vi "STAV Programs read_write.vi"() -> ()   [LabVIEW 2021]
uses:
  Czytaj RS/Biblioteki/Statyw/Application.ctl
  Czytaj RS/Biblioteki/Statyw/STAV CommandList.ctl
  Czytaj RS/Biblioteki/Statyw/STAV lib.lvlib
panel:
  out "String":string
  in  "stop":bool
  in  "Tab Control":enum32{"Konfig", "Page 2", "Help", "Debug"}(tab)
  in  "STAV com port":refnum<visa-resource-name>="COM4"
  in  "Refresh":bool
  in  "Set Active":bool
  in  "Dane":i32(listbox)
  in  "Pobierz":bool
  in  "NO":u8=1 min=1 max=50 step=1
  in  "Application":T1
  in  "Run app":bool
  in  "Stop app":bool
  in  "Reset app":bool
  in  "check active":bool
  out "Profile":string
  out "Steps":i32
  out "Step":string
  # "Units: Metric, Imperial"
  # "Direction: Up, Down"
  # "Mode: Cycles, Time"
  # "Stop Condition:\nDuration, Distance, Position, F greater, F smaller, Break, Keep F"
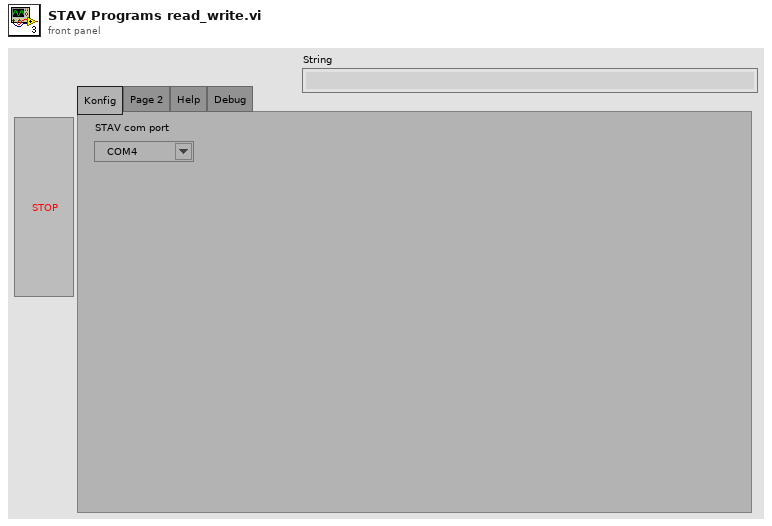
[diagram p1: front panel]
types:
  T1 = typedef "STAV lib.lvlib/Application.ctl" = enum16{"Peak", "Cycle", "Step", "Advanced"}
  T2 = enum8{"Enabled", "Disabled", "Disabled and Grayed Out"}
  T3 = typedef "STAV lib.lvlib/STAV CommandList.ctl" = enum16{"StartSending (0)", "StopSending(0)", "FindHomePos(0)", "SetSendingConfig(2)", "GetSendingConfig(0)", "SetPosition(2)", "SetSpeed(2)", "GetSpeed(0)", "GetPosition(0)", "GetForce(0)", "GetPeak(0)", "GetPeakDistance(0)", "GetTravelDistance(0)", "ResetTravelDistance(0)", "GetCycleNo(0)", "GetStepNo(0)", "GetDuration(0)", "GetProfilePosition(0)", "GetHoldTime(0)", "Stop(0)", "StartAndSend(0)", "Start(0)", "Reset(0)", "GetActiveProfile(0)", "SetActiveProfile(2)", "GetProfileCnt(1)", "GetMaxStepCnt(1)", "GetStepCnt(2)", "GetProfileIndex(2)", "SetProfile(3)", "SetStep(3+params)", "GetProfile(2)", "GetStep(3)", "SetProfile(2+params)", ""}
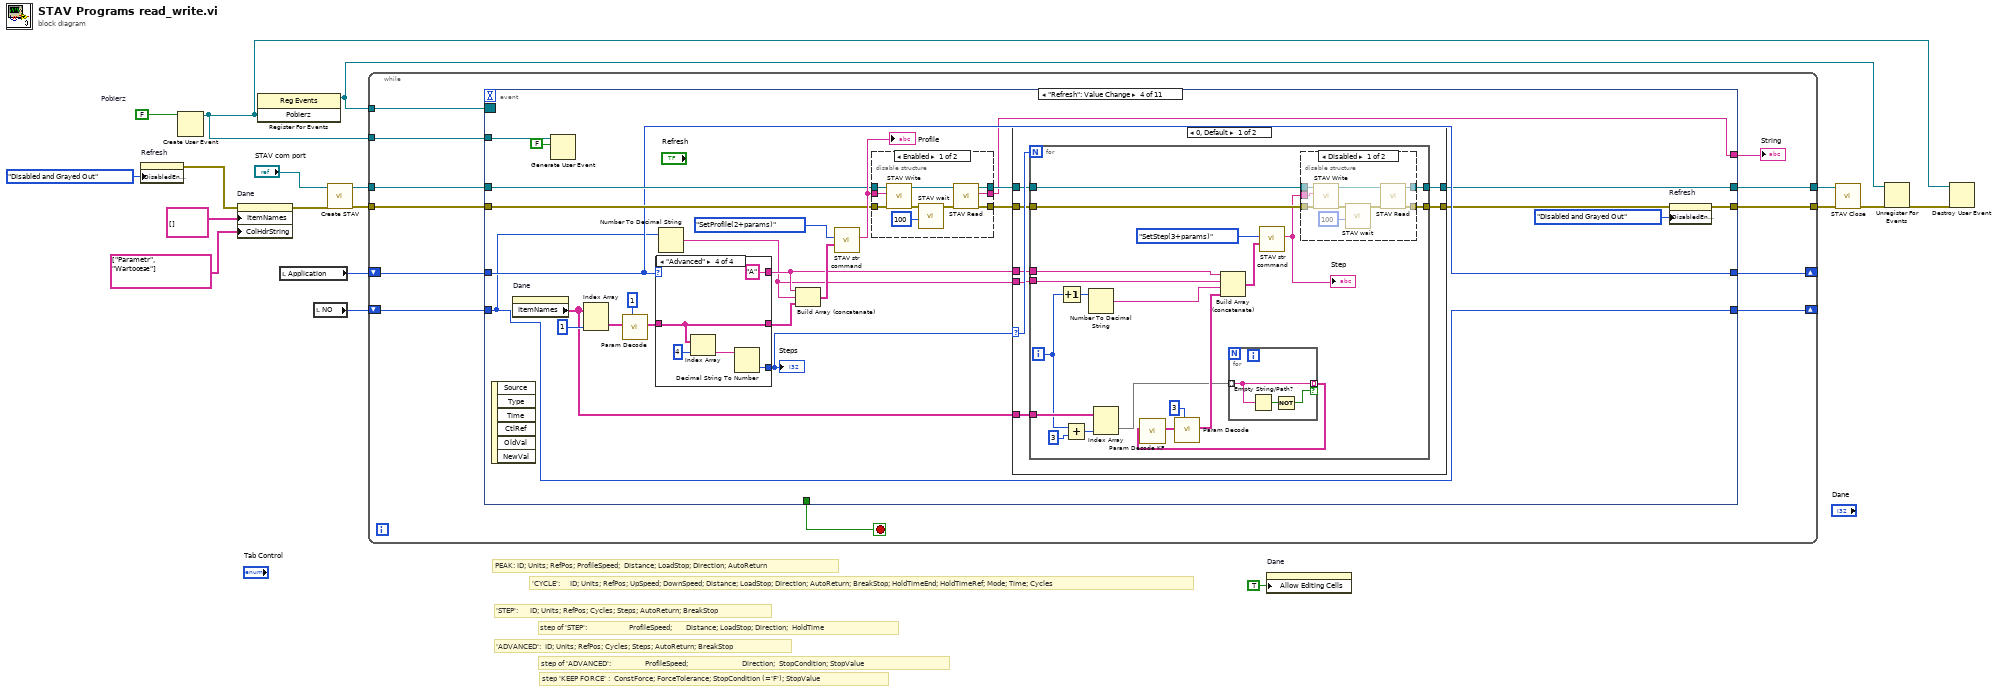
[diagram p0: block diagram]
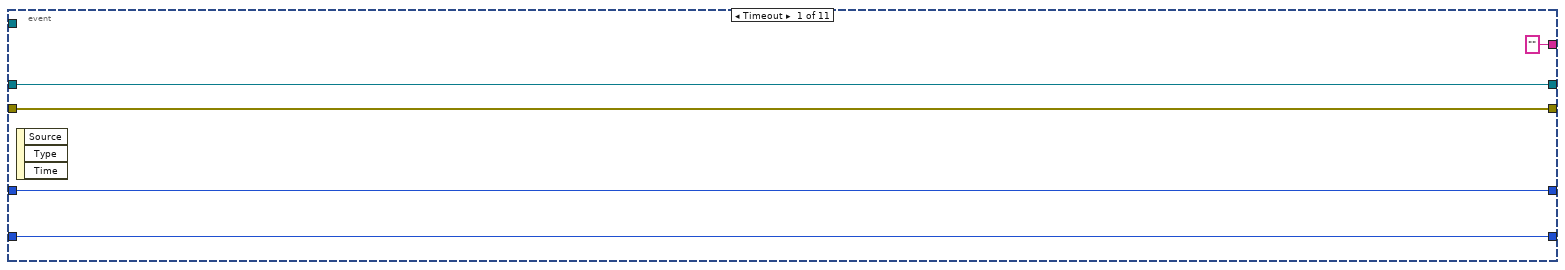
[diagram p2: hidden frame]
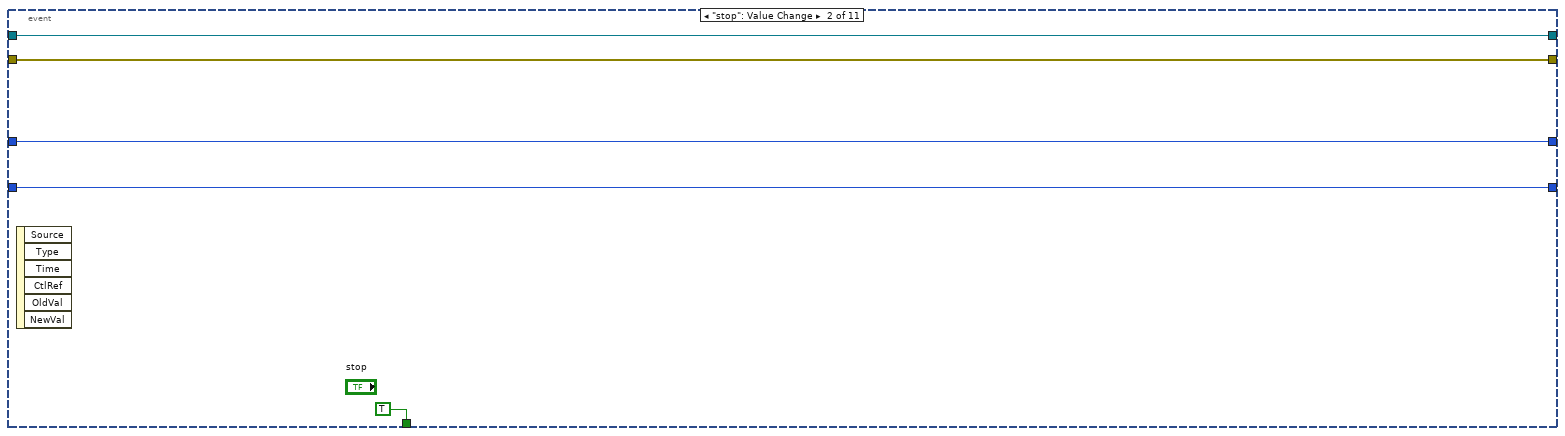
[diagram p3: hidden frame]
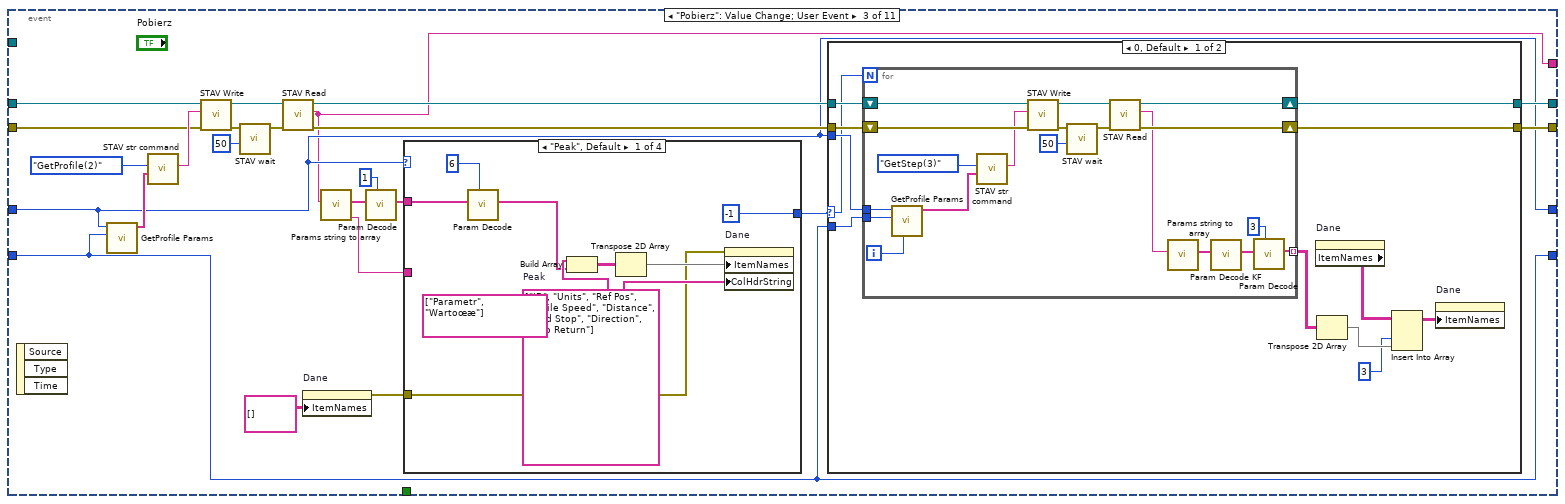
[diagram p4: hidden frame]
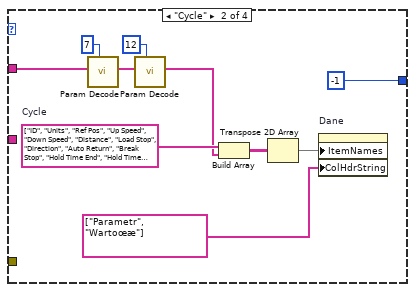
[diagram p6: hidden frame]
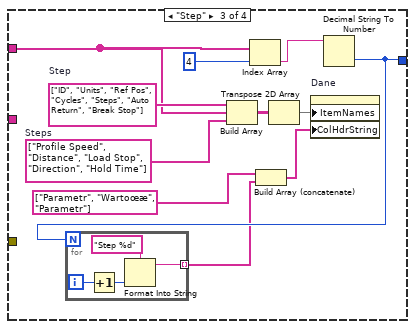
[diagram p7: hidden frame]
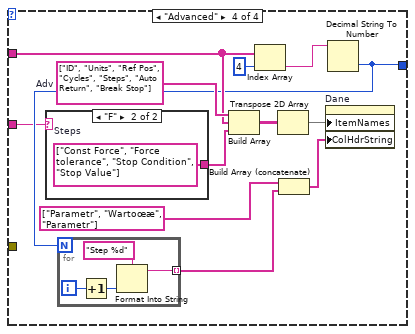
[diagram p8: hidden frame]
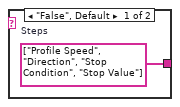
[diagram p9: hidden frame]
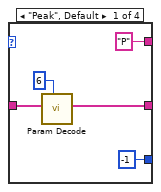
[diagram p13: hidden frame]
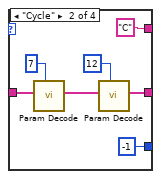
[diagram p14: hidden frame]
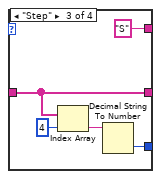
[diagram p15: hidden frame]
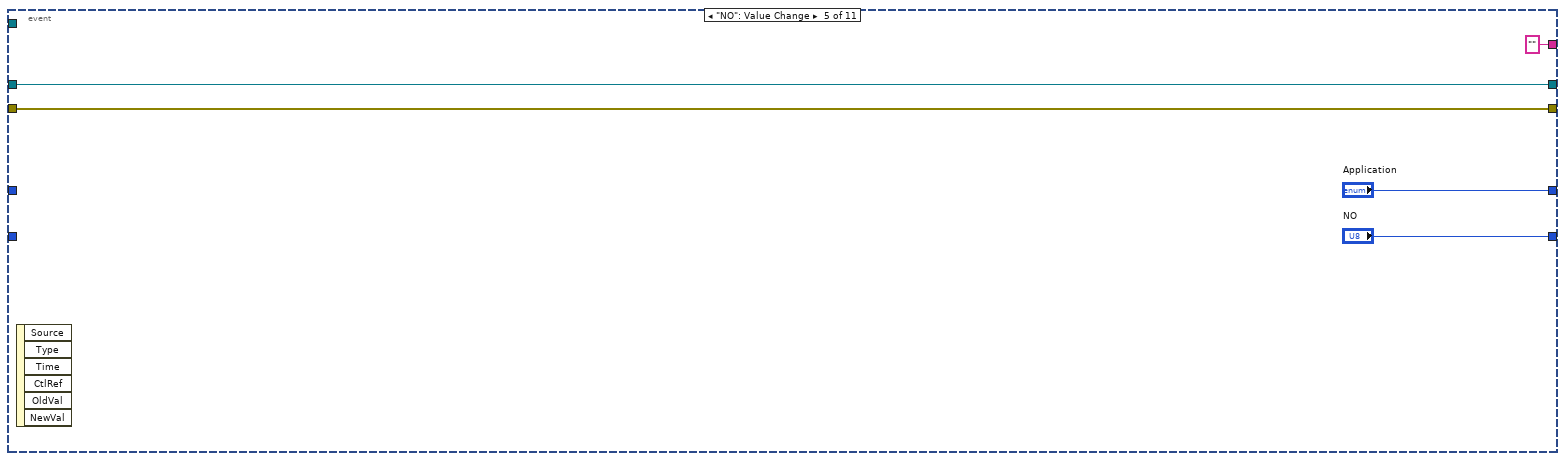
[diagram p16: hidden frame]
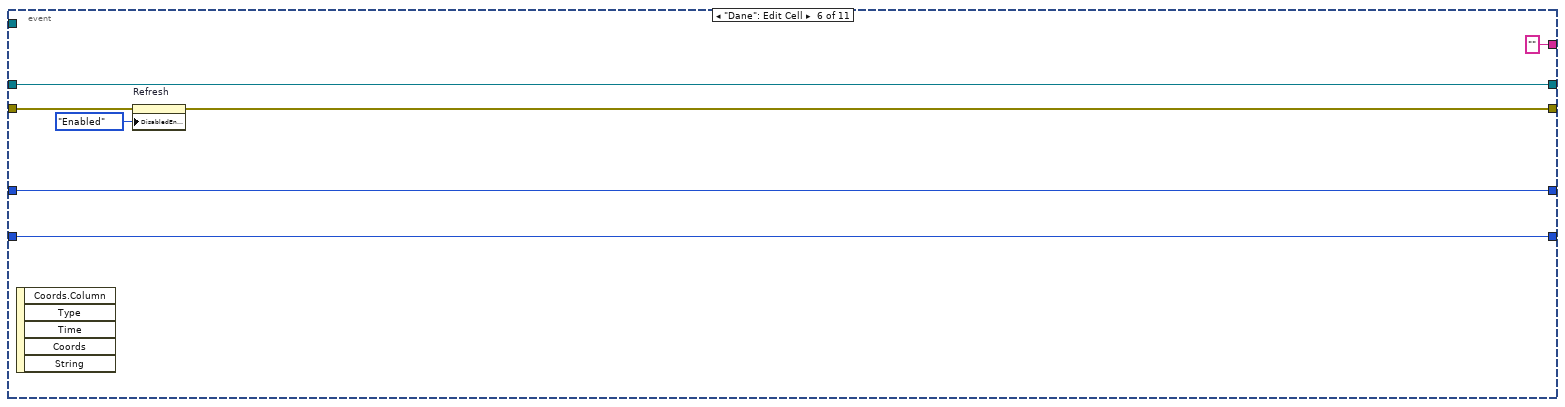
[diagram p17: hidden frame]
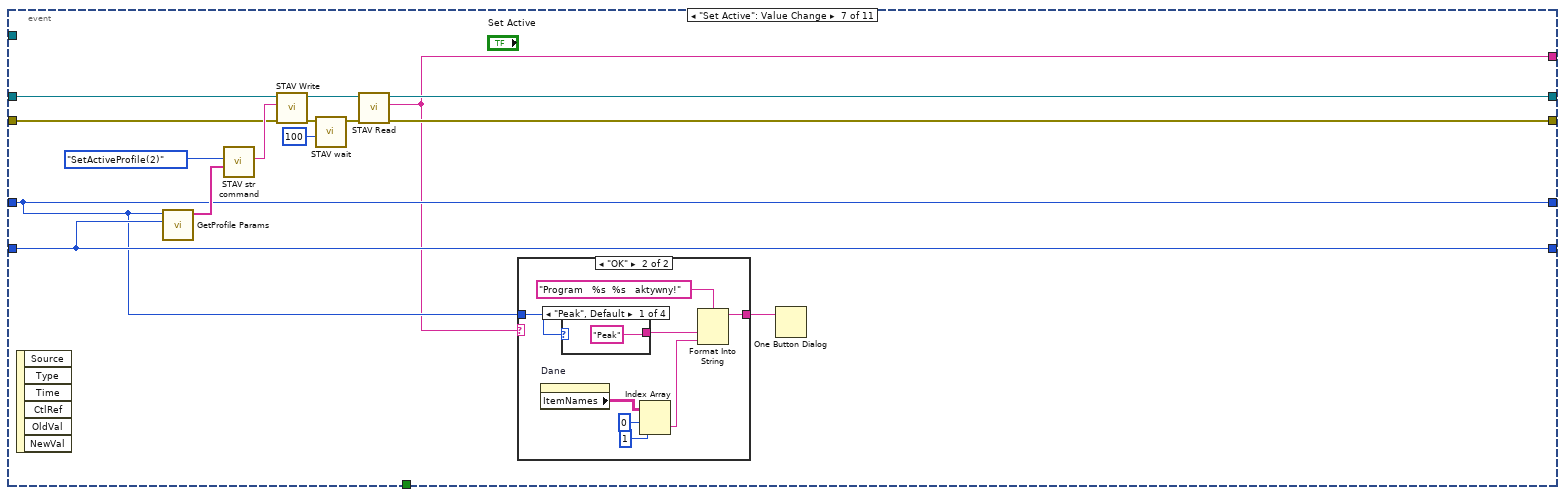
[diagram p18: hidden frame]
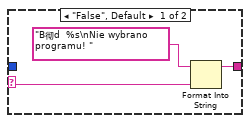
[diagram p19: hidden frame]
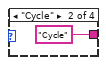
[diagram p20: hidden frame]
diagram:
  w5 = FALSE  # Pobierz
  # "step 'KEEP FORCE' :  ConstForce; ForceTolerance; StopCondition (='F'); StopValue"
  # "step of 'ADVANCED':                 ProfileSpeed;                           Direction;  StopCondition; StopValue"
  # "'ADVANCED':  ID; Units; RefPos; Cycles; Steps; AutoReturn; BreakStop"
  # "step of 'STEP':                     ProfileSpeed;       Distance; LoadStop; Direction;  HoldTime"
  # "'STEP':      ID; Units; RefPos; Cycles; Steps; AutoReturn; BreakStop"
  # "'CYCLE':     ID; Units; RefPos; UpSpeed; DownSpeed; Distance; LoadStop; Direction; AutoReturn; BreakStop; HoldTimeEnd; HoldTimeRef; Mode; Time; Cycles"
  # "PEAK: ID; Units; RefPos; ProfileSpeed;  Distance; LoadStop; Direction; AutoReturn"
  n1 = property on="Refresh" class="Bool"("DisabledEnum"=T2."Disabled and Grayed Out" ("Disabled")) -> (error out=w9:errorcluster)  [unwired: 2 in, 1 out]
  n2 = Create User Event(user event datatype=w5) -> (user event=w3:refnum<user-event>)  [unwired: 1 in, 1 out]
  n3 = property on="Dane" class="MCListbox (strict)"(error in=w9, "ItemNames"=string[][] [] ("Item Names"), "ColHdrString"=string[] ["Parametr", "Wartoœæ"] ("Column Header Strings[]")) -> (error out=w12:errorcluster)  [unwired: 1 in, 1 out]
  n4 = register-events(w3) -> (reference out=w4:refnum<event-registration>)  [unwired: 2 in, 1 out]
  n5 = local read "Application"() -> (w7:T1)
  n6 = local read "NO"() -> (w6:u8)
  n7 = call "Create STAV.vi"("error in (no error)"=w12, "STAV com port"="STAV com port") -> ("error out"=w16:errorcluster, "STAV ref out"=w17:refnum<visa-resource-name>)  [unwired: 8 in]
  n8 = while {
    tunnel: w17 -> [w29]
    tunnel: w16 -> [w28]
    tunnel: [w27] -> w15
    tunnel: [w26] -> w14
    shift-right: [w25] -> _
    shift-left: w7 -> [w23]
    shift-right: [w24] -> _
    shift-left: w6 -> [w22]
    tunnel: w4 -> [w21]
    tunnel: w3 -> [w20]
    stop <- w30 stop-if-true
    n9 = event shown="[3] \"Refresh\": Value Change" {
      selector: w21 -> [_ _ _ _ _ _ _ _ _ _ _]
      dyn-events: _ -> [_ _ _ _ _ _ _ _ _ _ _]
      timeout: _ -> [_ _ _ _ _ _ _ _ _ _ _]
      tunnel: [_ TRUE ("stop") _ _ _ _ _ _ _ _ _] -> w30
      tunnel: w29 -> [w35 w39 w61 w170 w252 w260 w270 w307 w330 w343 w356]
      tunnel: w28 -> [w34 w38 w60 w171 w253 w262 w271 w308 w329 w342 w355]
      tunnel: [w35 w39 w52 w155 w252 w260 w267 w304 w326 w339 w352] -> w27
      tunnel: [w34 w38 w50 w160 w253 w261 w268 w305 w327 w340 w353] -> w26
      tunnel: w22 -> [w32 w36 w45 w167 _ w258 w269 w306 w331 w344 w357]
      tunnel: w23 -> [w33 w37 w44 w168 _ w259 w265 w303 w332 w345 w358]
      tunnel: [w33 w37 w44 w168 "Application" w259 w265 w303 w332 w345 w358] -> w25
      tunnel: [w32 w36 w45 w167 "NO" w258 w269 w306 w331 w344 w357] -> w24
      tunnel: w20 -> [_ _ _ w151 _ _ _ _ _ _ _]
      tunnel: ["" ("String") _ w41 w149 "" ("String") "" ("String") w264 w294 w320 w333 w346] -> w19
      event Timeout {
        n10 = event-data() -> ()  [unwired: 1 in, 3 out]
      }
      event "stop": Value Change {
        n11 = event-data() -> ()  [unwired: 1 in, 6 out]
      }
      event "Pobierz": Value Change; User Event {
        n12 = event-data() -> ()  [unwired: 1 in, 3 out]
        n13 = call "GetProfile Params.vi"("NO"=w45, "Application"=w44) -> ("params array out"=w57:string[])  [unwired: 7 in, 2 out]
        n14 = call "STAV str command.vi"("Params"=w57, "Command"=STAV_CommandList."GetProfile(2)") -> ("str command"=w63:string)  [unwired: 8 in, 1 out]
        n15 = call "STAV Write.vi"("error in (no error)"=w60, "Command"=w63, "STAV ref in"=w61) -> ("error out"=w58:errorcluster, "STAV ref out"=w59:refnum<visa-resource-name>)  [unwired: 7 in]
        n16 = call "STAV wait.vi"("delay (20)"=u32 50, "error in (no error)"=w58) -> ("error out"=w56:errorcluster)  [unwired: 9 in]
        n17 = call "STAV Read.vi"("error in (no error)"=w56, "STAV ref in"=w59) -> ("error out"=w51:errorcluster, "String"=w41:string, "STAV ref out"=w53:refnum<visa-resource-name>)  [unwired: 6 in, 1 out]
        n18 = property on="Dane" class="MCListbox (strict)"("ItemNames"=string[][] [] ("Item Names")) -> (error out=w42:errorcluster)  [unwired: 2 in, 1 out]
        n19 = call "Params string to array.vi"("String params"=w41) -> ("Last"=w49:string, "Array of params"=w47:string[])  [unwired: 9 in]
        n20 = call "Param Decode.vi"("index"=1, "Array - letter"=w47) -> ("Array -parameter"=w46:string[])  [unwired: 8 in, 1 out]
        n21 = case shown="\"Peak\", Default" w44 {
          tunnel: w46 -> [w100 w110 w116 w138]
          tunnel: [-1 -1 w119 w135] -> w54
          tunnel: w49 -> [_ _ _ w131]
          tunnel: w42 -> [w97 _ _ _]
          frame "Peak", Default {
            w105 = string[] ["ID", "Units", "Ref Pos", "Profile Speed", "Distance", "Load Stop", "Direction", "Auto Return"]  # Peak
            n22 = call "Param Decode.vi"("index"=6, "Array - letter"=w100) -> ("Array -parameter"=w99:string[])  [unwired: 8 in, 1 out]
            n23 = Build Array(w105, w99) -> (w104:string[][])
            n24 = Transpose 2D Array(2D array=w104) -> (transposed array=w103:string[][])
            n25 = property on="Dane" class="MCListbox (strict)"(error in=w97, "ItemNames"=w103, "ColHdrString"=string[] ["Parametr", "Wartoœæ"] ("Column Header Strings[]")) -> ()  [unwired: 1 in, 2 out]
          }
          frame "Cycle" {
            w114 = string[] ["ID", "Units", "Ref Pos", "Up Speed", "Down Speed", "Distance", "Load Stop", "Direction", "Auto Return", "Break Stop", "Hold Time End", "Hold Time Ref", "Mode", "Time", "Cycles"]  # Cycle
            n26 = call "Param Decode.vi"("index"=7, "Array - letter"=w110) -> ("Array -parameter"=w107:string[])  [unwired: 8 in, 1 out]
            n27 = call "Param Decode.vi"("index"=12, "Array - letter"=w107) -> ("Array -parameter"=w106:string[])  [unwired: 8 in, 1 out]
            n28 = Build Array(w114, w106) -> (w115:string[][])
            n29 = Transpose 2D Array(2D array=w115) -> (transposed array=w113:string[][])
            n30 = property on="Dane" class="MCListbox (strict)"("ItemNames"=w113, "ColHdrString"=string[] ["Parametr", "Wartoœæ"] ("Column Header Strings[]")) -> ()  [unwired: 2 in, 2 out]
          }
          frame "Step" {
            w117 = string[] ["Profile Speed", "Distance", "Load Stop", "Direction", "Hold Time"]  # Steps
            w124 = string[] ["ID", "Units", "Ref Pos", "Cycles", "Steps", "Auto Return", "Break Stop"]  # Step
            n31 = Build Array(w124, w116, w117) -> (w126:string[][])
            n32 = Index Array(array=w116, index=4) -> (element=w122:string)
            n33 = Transpose 2D Array(2D array=w126) -> (transposed array=w125:string[][])
            n34 = Decimal String To Number(string=w122) -> (number=w119:i32)  [unwired: 2 in, 1 out]
            n35 = for {
              N: w119 -> [_]
              tunnel: [w128] -> w118 mode=indexing
              i -> [w130]
              n36 = Increment(x=w130) -> (x+1=w127:i32)
              n37 = Format Into String(format string="Step %d", w127) -> (resulting string=w128:string)  [unwired: 2 in, 1 out]
            }
            n38 = Build Array (concatenate)(string[] ["Parametr", "Wartoœæ", "Parametr"] ("Column Header Strings[]"), w118) -> (w120:string[])
            n39 = property on="Dane" class="MCListbox (strict)"("ItemNames"=w125, "ColHdrString"=w120) -> ()  [unwired: 2 in, 2 out]
          }
          frame "Advanced" {
            w139 = string[] ["ID", "Units", "Ref Pos", "Cycles", "Steps", "Auto Return", "Break Stop"]  # Adv
            n40 = case shown="\"F\"" w131 {
              tunnel: [w143 w144] -> w132
              frame "False", Default {
                w143 = string[] ["Profile Speed", "Direction", "Stop Condition", "Stop Value"]  # Steps
              }
              frame "F" {
                w144 = string[] ["Const Force", "Force tolerance", "Stop Condition", "Stop Value"]  # Steps
              }
            }
            n41 = Build Array(w139, w138, w132) -> (w142:string[][])
            n42 = Index Array(array=w138, index=4) -> (element=w136:string)
            n43 = Transpose 2D Array(2D array=w142) -> (transposed array=w141:string[][])
            n44 = Decimal String To Number(string=w136) -> (number=w135:i32)  [unwired: 2 in, 1 out]
            n45 = for {
              N: w135 -> [_]
              tunnel: [w146] -> w133 mode=indexing
              i -> [w148]
              n46 = Increment(x=w148) -> (x+1=w145:i32)
              n47 = Format Into String(format string="Step %d", w145) -> (resulting string=w146:string)  [unwired: 2 in, 1 out]
            }
            n48 = Build Array (concatenate)(string[] ["Parametr", "Wartoœæ", "Parametr"] ("Column Header Strings[]"), w133) -> (w134:string[])
            n49 = property on="Dane" class="MCListbox (strict)"("ItemNames"=w141, "ColHdrString"=w134) -> ()  [unwired: 2 in, 2 out]
          }
        }
        n50 = case shown="0, Default" w54 {
          selector: w54 -> [w69 _]
          tunnel: w53 -> [w74 w96]
          tunnel: [w72 w96] -> w52
          tunnel: w51 -> [w75 w95]
          tunnel: [w73 w95] -> w50
          tunnel: w44 -> [w71 _]
          tunnel: w45 -> [w70 _]
          frame 0, Default {
            n51 = for {
              N: w69 -> [_]
              shift-right: [w87] -> w73
              shift-left: w75 -> [w89]
              shift-right: [w86] -> w72
              shift-left: w74 -> [w88]
              tunnel: w71 -> [w84]
              tunnel: w70 -> [w83]
              tunnel: [w78] -> w68 mode=indexing
              i -> [w80]
              n52 = call "GetProfile Params.vi"("Step (-1)"=w80, "NO"=w83, "Application"=w84) -> ("params array out"=w82:string[])  [unwired: 6 in, 2 out]
              n53 = call "STAV str command.vi"("Params"=w82, "Command"=STAV_CommandList."GetStep(3)") -> ("str command"=w85:string)  [unwired: 8 in, 1 out]
              n54 = call "STAV Write.vi"("error in (no error)"=w89, "Command"=w85, "STAV ref in"=w88) -> ("error out"=w91:errorcluster, "STAV ref out"=w90:refnum<visa-resource-name>)  [unwired: 7 in]
              n55 = call "STAV wait.vi"("delay (20)"=u32 50, "error in (no error)"=w91) -> ("error out"=w92:errorcluster)  [unwired: 9 in]
              n56 = call "STAV Read.vi"("error in (no error)"=w92, "STAV ref in"=w90) -> ("error out"=w87:errorcluster, "String"=w81:string, "STAV ref out"=w86:refnum<visa-resource-name>)  [unwired: 6 in, 1 out]
              n57 = call "Params string to array.vi"("String params"=w81) -> ("Array of params"=w77:string[])  [unwired: 9 in, 1 out]
              n58 = call "Param Decode KF.vi"("Array - letter"=w77) -> ("Array -parameter"=w76:string[])  [unwired: 9 in, 1 out]
              n59 = call "Param Decode.vi"("index"=3, "Array - letter"=w76) -> ("Array -parameter"=w78:string[])  [unwired: 8 in, 1 out]
            }
            n60 = property on="Dane" class="MCListbox (strict)"() -> ("ItemNames"=w67:string[][])  [unwired: 2 in, 2 out]
            n61 = Transpose 2D Array(2D array=w68) -> (transposed array=w65:string[][])
            n62 = Insert Into Array(array=w67, index (col)=3 ("disabled index (col)"), new element=w65) -> (w66:string[][])  [unwired: 1 in]
            n63 = property on="Dane" class="MCListbox (strict)"("ItemNames"=w66) -> ()  [unwired: 2 in, 2 out]
          }
          frame -1 {
          }
        }
      }
      event "Refresh": Value Change {
        n64 = event-data() -> ()  [unwired: 1 in, 6 out]
        n65 = property on="Dane" class="MCListbox (strict)"() -> ("ItemNames"=w154:string[][])  [unwired: 2 in, 2 out]
        n66 = Generate User Event(user event=w151, event data cluster=FALSE ("event data")) -> ()  [unwired: 2 in, 2 out]
        n67 = Index Array(array=w154, index (col)=1 ("disabled index (col)")) -> (element=w164:string[])  [unwired: 1 in]
        n68 = call "Param Decode.vi"("index"=1, "Array - letter"=w164) -> ("Array -parameter"=w163:string[])  [unwired: 8 in, 1 out]
        n69 = case shown="\"Advanced\"" w168 {
          tunnel: ["P" "C" "S" "A"] -> w153
          tunnel: w163 -> [w233 w240 w245 w249]
          tunnel: [w232 w237 w245 w249] -> w165
          tunnel: [-1 -1 w242 w247] -> w159
          frame "Peak", Default {
            n70 = call "Param Decode.vi"("index"=6, "Array - letter"=w233) -> ("Array -parameter"=w232:string[])  [unwired: 8 in, 1 out]
          }
          frame "Cycle" {
            n71 = call "Param Decode.vi"("index"=7, "Array - letter"=w240) -> ("Array -parameter"=w238:string[])  [unwired: 8 in, 1 out]
            n72 = call "Param Decode.vi"("index"=12, "Array - letter"=w238) -> ("Array -parameter"=w237:string[])  [unwired: 8 in, 1 out]
          }
          frame "Step" {
            n73 = Index Array(array=w245, index=4) -> (element=w243:string)
            n74 = Decimal String To Number(string=w243) -> (number=w242:i32)  [unwired: 2 in, 1 out]
          }
          frame "Advanced" {
            n75 = Index Array(array=w249, index=4) -> (element=w248:string)
            n76 = Decimal String To Number(string=w248) -> (number=w247:i32)  [unwired: 2 in, 1 out]
          }
        }
        "Steps" <- w159
        n77 = Number To Decimal String(number=w167) -> (decimal integer string=w152:string)  [unwired: 1 in]
        n78 = Build Array (concatenate)(w153, w152, w165) -> (w166:string[])
        n79 = call "STAV str command.vi"("Params"=w166, "Command"=STAV_CommandList."SetProfile(2+params)") -> ("str command"=w173:string)  [unwired: 8 in, 1 out]
        "Profile" <- w173
        n80 = disable-structure shown="Enabled" {
          disable-tunnel: w173 -> [w227 _]
          disable-tunnel: w171 -> [w222 w228]
          disable-tunnel: w170 -> [w221 w229]
          disable-tunnel: [w220 w228] -> w157
          disable-tunnel: [w219 w229] -> w158
          disable-tunnel: [w218 _] -> w149
          frame Enabled {
            n81 = call "STAV Write.vi"("error in (no error)"=w222, "Command"=w227, "STAV ref in"=w221) -> ("error out"=w225:errorcluster, "STAV ref out"=w226:refnum<visa-resource-name>)  [unwired: 7 in]
            n82 = call "STAV wait.vi"("delay (20)"=u32 100, "error in (no error)"=w225) -> ("error out"=w224:errorcluster)  [unwired: 9 in]
            n83 = call "STAV Read.vi"("error in (no error)"=w224, "STAV ref in"=w226) -> ("error out"=w220:errorcluster, "String"=w218:string, "STAV ref out"=w219:refnum<visa-resource-name>)  [unwired: 6 in, 1 out]
          }
          frame Disabled {
          }
        }
        n84 = case shown="0, Default" w159 {
          selector: w159 -> [w181 _]
          tunnel: w158 -> [w180 w216]
          tunnel: w157 -> [w179 w217]
          tunnel: [w178 w217] -> w156
          tunnel: [w177 w216] -> w155
          tunnel: w154 -> [w176 _]
          tunnel: w153 -> [w175 _]
          tunnel: w152 -> [w174 _]
          frame 0, Default {
            n85 = for {
              N: w181 -> [_]
              tunnel: w180 -> [w200]
              tunnel: w179 -> [w199]
              tunnel: [w198] -> w178
              tunnel: [w197] -> w177
              tunnel: w176 -> [w196]
              tunnel: w175 -> [w195]
              tunnel: w174 -> [w194]
              i -> [w191]
              n86 = Increment(x=w191) -> (x+1=w193:i32)
              n87 = Add(x=w191, y=3) -> (x+y=w184:i32)
              n88 = Number To Decimal String(number=w193) -> (decimal integer string=w192:string)  [unwired: 1 in]
              n89 = Index Array(array=w196, index (col)=w184) -> (element=w183:string[])  [unwired: 1 in]
              n90 = for {
                tunnel: w183 -> [w204] mode=indexing
                tunnel: [w204] -> w182 mode=indexing if=w202
                n91 = Empty String/Path?(string/path=w204) -> (empty?=w203:bool)
                n92 = Not(x=w203) -> (.not. x?=w202:bool)
              }
              n93 = call "Param Decode KF.vi"("Array - letter"=w182) -> ("Array -parameter"=w186:string[])  [unwired: 9 in, 1 out]
              n94 = call "Param Decode.vi"("index"=3, "Array - letter"=w186) -> ("Array -parameter"=w185:string[])  [unwired: 8 in, 1 out]
              n95 = Build Array (concatenate)(w195, w194, w192, w185) -> (w189:string[])
              n96 = call "STAV str command.vi"("Params"=w189, "Command"=STAV_CommandList."SetStep(3+params)") -> ("str command"=w188:string)  [unwired: 8 in, 1 out]
              "Step" <- w188
              n97 = disable-structure shown="Disabled" {
                disable-tunnel: w200 -> [w209 w215]
                disable-tunnel: w199 -> [w208 w214]
                disable-tunnel: [w207 w214] -> w198
                disable-tunnel: [w206 w215] -> w197
                disable-tunnel: w188 -> [w205 _]
                frame Disabled {
                  n98 = call "STAV Write.vi"("error in (no error)"=w208, "Command"=w205, "STAV ref in"=w209) -> ("error out"=w211:errorcluster, "STAV ref out"=w210:refnum<visa-resource-name>)  [unwired: 7 in]
                  n99 = call "STAV wait.vi"("delay (20)"=u32 100, "error in (no error)"=w211) -> ("error out"=w212:errorcluster)  [unwired: 9 in]
                  n100 = call "STAV Read.vi"("error in (no error)"=w212, "STAV ref in"=w210) -> ("error out"=w207:errorcluster, "STAV ref out"=w206:refnum<visa-resource-name>)  [unwired: 6 in, 2 out]
                }
                frame Enabled {
                }
              }
            }
          }
          frame -1 {
          }
        }
        n101 = property on="Refresh" class="Bool"(error in=w156, "DisabledEnum"=T2."Disabled and Grayed Out" ("Disabled")) -> (error out=w160:errorcluster)  [unwired: 1 in, 1 out]
      }
      event "NO": Value Change {
        n102 = event-data() -> ()  [unwired: 1 in, 6 out]
      }
      event "Dane": Edit Cell {
        n103 = event-data() -> ()  [unwired: 1 in, 5 out]
        n104 = property on="Refresh" class="Bool"(error in=w262, "DisabledEnum"=T2."Enabled" ("Disabled")) -> (error out=w261:errorcluster)  [unwired: 1 in, 1 out]
      }
      event "Set Active": Value Change {
        n105 = event-data() -> ()  [unwired: 1 in, 6 out]
        n106 = call "GetProfile Params.vi"("NO"=w269, "Application"=w265) -> ("params array out"=w274:string[])  [unwired: 7 in, 2 out]
        n107 = call "STAV str command.vi"("Params"=w274, "Command"=STAV_CommandList."SetActiveProfile(2)") -> ("str command"=w278:string)  [unwired: 8 in, 1 out]
        n108 = call "STAV Write.vi"("error in (no error)"=w271, "Command"=w278, "STAV ref in"=w270) -> ("error out"=w275:errorcluster, "STAV ref out"=w276:refnum<visa-resource-name>)  [unwired: 7 in]
        n109 = call "STAV wait.vi"("delay (20)"=u32 100, "error in (no error)"=w275) -> ("error out"=w273:errorcluster)  [unwired: 9 in]
        n110 = call "STAV Read.vi"("error in (no error)"=w273, "STAV ref in"=w276) -> ("error out"=w268:errorcluster, "String"=w264:string, "STAV ref out"=w267:refnum<visa-resource-name>)  [unwired: 6 in, 1 out]
        n111 = case shown="\"OK\"" w264 {
          selector: w264 -> [w280 _]
          tunnel: [w279 w285] -> w266
          tunnel: w265 -> [_ w284]
          frame "False", Default {
            n112 = Format Into String(initial string="B彻d  %s\nNie wybrano programu! ", w280) -> (resulting string=w279:string)  [unwired: 2 in, 1 out]
          }
          frame "OK" {
            n113 = property on="Dane" class="MCListbox (strict)"() -> ("ItemNames"=w289:string[][])  [unwired: 2 in, 2 out]
            n114 = case shown="\"Peak\", Default" w284 {
              tunnel: ["Peak" ("format string") "Cycle" ("format string") "Step" ("format string") "Advanced" ("format string")] -> w282
              frame "Peak", Default {
              }
              frame "Cycle" {
              }
              frame "Step" {
              }
              frame "Advanced" {
              }
            }
            n115 = Index Array(array=w289, index (row)=0, index (col)=1 ("disabled index (col)")) -> (element=w283:string)
            n116 = Format Into String(format string="Program   %s  %s   aktywny!", w282, w283) -> (resulting string=w285:string)  [unwired: 2 in, 1 out]
          }
        }
        n117 = One Button Dialog(message=w266) -> ()  [unwired: 1 in, 1 out]
      }
      event "check active": Value Change {
        n118 = event-data() -> ()  [unwired: 1 in, 6 out]
        n119 = call "STAV str command.vi"("Command"=STAV_CommandList."GetActiveProfile(0)") -> ("str command"=w314:string)  [unwired: 9 in, 1 out]
        n120 = call "STAV Write.vi"("error in (no error)"=w308, "Command"=w314, "STAV ref in"=w307) -> ("error out"=w311:errorcluster, "STAV ref out"=w312:refnum<visa-resource-name>)  [unwired: 7 in]
        n121 = call "STAV wait.vi"("delay (20)"=u32 100, "error in (no error)"=w311) -> ("error out"=w310:errorcluster)  [unwired: 9 in]
        n122 = call "STAV Read.vi"("error in (no error)"=w310, "STAV ref in"=w312) -> ("error out"=w305:errorcluster, "String"=w294:string, "STAV ref out"=w304:refnum<visa-resource-name>)  [unwired: 6 in, 1 out]
        n123 = String Subset(string=w294, offset (0)=0, length (rest)=1 ("length (rest)")) -> (substring=w299:string)
        n124 = String Subset(string=w294, offset (0)=2) -> (substring=w295:string)  [unwired: 1 in]
        n125 = case shown="\"False\", Default" w299 {
          tunnel: ["- brak -" ("substring") "Peak" ("substring") "Cycle" ("substring") "Step" ("substring") "Advanced" ("substring")] -> w296
          frame "False", Default {
          }
          frame "P" {
          }
          frame "C" {
          }
          frame "S" {
          }
          frame "A" {
          }
        }
        n126 = Format Into String(format string="Aktywny program \\n\n%s , numer %s", w296, w295) -> (resulting string=w297:string)  [unwired: 2 in, 1 out]
        n127 = One Button Dialog(message=w297) -> ()  [unwired: 1 in, 1 out]
      }
      event "Run app": Value Change {
        n128 = event-data() -> ()  [unwired: 1 in, 6 out]
        n129 = call "STAV str command.vi"("Command"=STAV_CommandList."Start(0)") -> ("str command"=w322:string)  [unwired: 9 in, 1 out]
        n130 = call "STAV Write.vi"("error in (no error)"=w329, "Command"=w322, "STAV ref in"=w330) -> ("error out"=w325:errorcluster, "STAV ref out"=w328:refnum<visa-resource-name>)  [unwired: 7 in]
        n131 = call "STAV wait.vi"("delay (20)"=u32 100, "error in (no error)"=w325) -> ("error out"=w324:errorcluster)  [unwired: 9 in]
        n132 = call "STAV Read.vi"("error in (no error)"=w324, "STAV ref in"=w328) -> ("error out"=w327:errorcluster, "String"=w320:string, "STAV ref out"=w326:refnum<visa-resource-name>)  [unwired: 6 in, 1 out]
      }
      event "Stop app": Value Change {
        n133 = event-data() -> ()  [unwired: 1 in, 6 out]
        n134 = call "STAV str command.vi"("Command"=STAV_CommandList."Stop(0)") -> ("str command"=w335:string)  [unwired: 9 in, 1 out]
        n135 = call "STAV Write.vi"("error in (no error)"=w342, "Command"=w335, "STAV ref in"=w343) -> ("error out"=w338:errorcluster, "STAV ref out"=w341:refnum<visa-resource-name>)  [unwired: 7 in]
        n136 = call "STAV wait.vi"("delay (20)"=u32 100, "error in (no error)"=w338) -> ("error out"=w337:errorcluster)  [unwired: 9 in]
        n137 = call "STAV Read.vi"("error in (no error)"=w337, "STAV ref in"=w341) -> ("error out"=w340:errorcluster, "String"=w333:string, "STAV ref out"=w339:refnum<visa-resource-name>)  [unwired: 6 in, 1 out]
      }
      event "Reset app": Value Change {
        n138 = event-data() -> ()  [unwired: 1 in, 6 out]
        n139 = call "STAV str command.vi"("Command"=STAV_CommandList."Reset(0)") -> ("str command"=w348:string)  [unwired: 9 in, 1 out]
        n140 = call "STAV Write.vi"("error in (no error)"=w355, "Command"=w348, "STAV ref in"=w356) -> ("error out"=w351:errorcluster, "STAV ref out"=w354:refnum<visa-resource-name>)  [unwired: 7 in]
        n141 = call "STAV wait.vi"("delay (20)"=u32 100, "error in (no error)"=w351) -> ("error out"=w350:errorcluster)  [unwired: 9 in]
        n142 = call "STAV Read.vi"("error in (no error)"=w350, "STAV ref in"=w354) -> ("error out"=w353:errorcluster, "String"=w346:string, "STAV ref out"=w352:refnum<visa-resource-name>)  [unwired: 6 in, 1 out]
      }
    }
    "String" <- w19
  }
  n143 = property on="Dane" class="MCListbox (strict)"("Allow Editing Cells"=TRUE) -> ()  [unwired: 2 in, 2 out]
  n144 = call "STAV Close.vi"("error in (no error)"=w14, "STAV ref in"=w15) -> ("error out"=w1:errorcluster)  [unwired: 9 in]
  n145 = Unregister For Events(event registration refnum=w4, error in=w1) -> (error out=w2:errorcluster)
  n146 = Destroy User Event(user event=w3, error in=w2) -> ()  [unwired: 1 out]
